vi "Flow rate calc_Druck.vi"(9 "T venturi":fxp<+/-,42,16> format="%.31g", 10 "P venturi":fxp<+/-,42,16> format="%.31g") -> (1 "Flow rate g/s":dbl, 2 "Flow rate l/min":dbl)   [LabVIEW 2014]
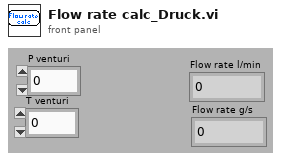
[diagram p1: front panel]
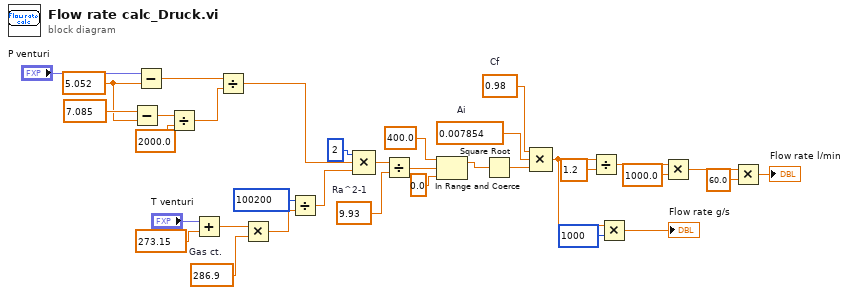
[diagram p0: block diagram]
diagram:
  w28 = 9.93  # Ra^2-1
  w25 = 0.98  # Cf
  w6 = 5.052
  w31 = 286.9  # Gas ct.
  w26 = 0.007854  # Ai
  n1 = Subtract(x=7.085, y=w6) -> (x-y=w5:dbl)
  n2 = Subtract(x="P venturi", y=w6) -> (x-y=w2:dbl)
  n3 = Divide(x=w5, y=2000.0) -> (x/y=w3:dbl)
  n4 = Add(x="T venturi", y=273.15) -> (x+y=w32:dbl)
  n5 = Divide(x=w2, y=w3) -> (x/y=w1:dbl)
  n6 = Multiply(x=w32, y=w31) -> (x*y=w23:dbl)
  n7 = Divide(x=100200, y=w23) -> (x/y=w22:dbl)
  n8 = Compound Arithmetic op=MULTIPLY(2, w1, w22) -> (w29:dbl)
  n9 = Divide(x=w29, y=w28) -> (x/y=w12:dbl)
  n10 = In Range and Coerce(upper limit=400.0, x=w12, lower limit=0.0) -> (coerced(x)=w9:dbl)  [unwired: 1 out]
  n11 = Square Root(x=w9) -> (sqrt(x)=w27:dbl)
  n12 = Compound Arithmetic op=MULTIPLY(w25, w26, w27) -> (w19:dbl)
  n13 = Divide(x=w19, y=1.2) -> (x/y=w17:dbl)
  n14 = Multiply(x=w19, y=1000) -> (x*y=→"Flow rate g/s":dbl)
  n15 = Multiply(x=w17, y=1000.0) -> (x*y=w15:dbl)
  n16 = Multiply(x=w15, y=60.0) -> (x*y=→"Flow rate l/min":dbl)
